vi "pmu_Write CFG Frame Type.vi"(8 "error in (no error)":errorcluster, 10 "configuration frame option":T1, 11 "system info in":refnum<class "PMU System Info.lvclass">) -> (0 "error out":errorcluster, 3 "system info out":refnum<class "PMU System Info.lvclass">)   [LabVIEW 2013, in "NI_EP_PMU.lvlib" / "PMU System Info.lvclass"]
uses:
  <vilib>/addons/Electrical Power/PMU/Common/Classes/PMU System Info/PMU System Info.lvclass
  <vilib>/addons/Electrical Power/PMU/Common/Controls/pmu_CFG for Data Frame.ctl
  <vilib>/addons/Electrical Power/PMU/Common/Classes/PMU System Info/PMU System Info.lvclass/PMU System Info.ctl
  <vilib>/addons/Electrical Power/PMU/NI_EP_PMU.lvlib
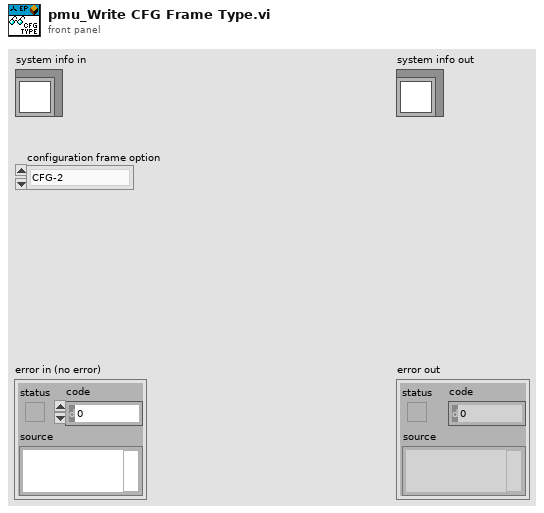
[diagram p1: front panel]
types:
  T1 = typedef "NI_EP_PMU.lvlib/pmu_CFG for Data Frame.ctl" = enum8{"CFG-2", "CFG-3", "CFG-2 and CFG-3"}
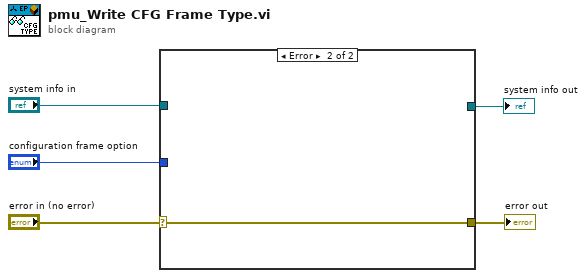
[diagram p0: block diagram]
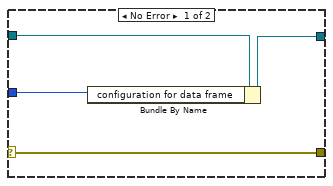
[diagram p2: hidden frame]
diagram:
  n1 = case shown="Error" "error in (no error)" {
    selector: "error in (no error)" -> [w9 w10]
    tunnel: "system info in" -> [w7 _]
    tunnel: [w9 w10] -> w3
    tunnel: "configuration frame option" -> [w8 _]
    tunnel: [w6 _] -> w1
    frame No Error {
      n2 = Bundle By Name(cluster=w7, "configuration for data frame"=w8) -> (w6:refnum<class "PMU System Info.lvclass">)
    }
    frame Error {
    }
  }
  "error out" <- w3
  "system info out" <- w1
